vi "WPI_DashboardGet Robot IP.vi"(11 "Notifier in":refnum<notifier>) -> ()   [LabVIEW 2018]
doc: "Connect to the Driver Station to receive occasional updates including the robot IP address. Send\nnotification when you receive IP information."
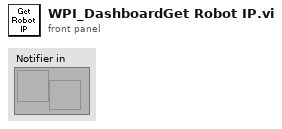
[diagram p1: front panel]
types:
  T1 = cluster{"robotIP":u32, "dashboardIP":u32, "FMS Connected":bool, "Robot Connected":bool, "RobotCode":bool}
  T2 = enum16{"Standard", "Buffered", "CRLF", "Immediate"}
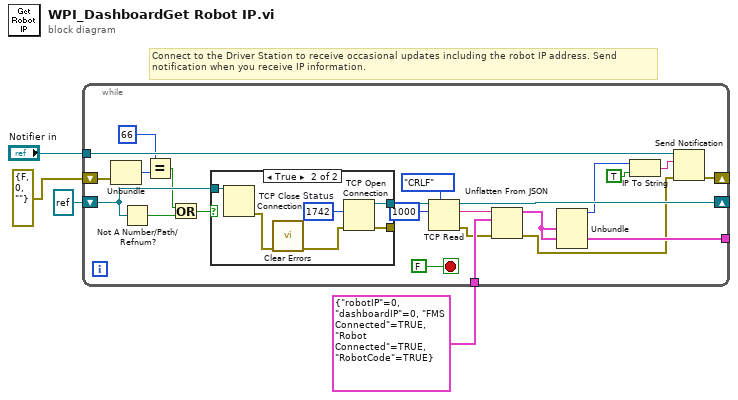
[diagram p0: block diagram]
diagram:
  # "Connect to the Driver Station to receive occasional updates including the robot IP address. Send\nnotification when you receive IP information."
  n1 = while {
    shift-right: [w22] -> _
    shift-left: refnum<k5> refnum ("connection ID") -> [w26]
    tunnel: [w18] -> _
    tunnel: T1 {"robotIP"=0, "dashboardIP"=0, "FMS Connected"=TRUE, "Robot Connected"=TRUE, "RobotCode"=TRUE} -> [w19]
    tunnel: "Notifier in" -> [w17]
    shift-right: [w11] -> _
    shift-left: errorcluster {"status"=FALSE, "code"=0, "source"=""} ("error out") -> [w8]
    stop <- FALSE stop-if-true
    n2 = Unbundle(w8) -> ("code"=w7:i32)  [unwired: 2 out]
    n3 = Not A Number/Path/Refnum?(number/path/refnum=w26) -> (NaN/Path/Refnum?=w10:bool)
    n4 = Equal?(x=66, y=w7) -> (x = y?=w5:bool)
    n5 = Or(x=w5, y=w10) -> (x .or. y?=w9:bool)
    n6 = case shown="True" w9 {
      tunnel: [w27 w32] -> w24
      tunnel: w26 -> [w27 w31]
      tunnel: [_ w30] -> _
      frame False {
      }
      frame True {
        w33 = u16 1742  # Status
        n7 = TCP Close Connection(connection ID=w31) -> (error out=w29:errorcluster)  [unwired: 2 in, 1 out]
        n8 = call <vilib>:"Clear Errors.vi"("error in (no error)"=w29) -> ("error out"=w28:errorcluster)  [unwired: 5 in, 1 out]
        n9 = TCP Open Connection(remote port or service name=w33, error in (no error)=w28) -> (connection ID=w32:refnum<k5>, error out=w30:errorcluster)  [unwired: 3 in]
      }
    }
    n10 = TCP Read(connection ID=w24, bytes to read=1000, 7:T2."CRLF" ("mode (standard)")) -> (connection ID out=w22:refnum<k5>, data out=w20:string, error out=w15:errorcluster)  [unwired: 2 in]
    n11 = Unflatten From JSON(JSON string=w20, type and defaults=w19, error in (no error)=w15) -> (value=w18:T1, error out=w12:errorcluster)  [unwired: 4 in]
    n12 = Unbundle(w18) -> ("robotIP"=w16:u32)  [unwired: 4 out]
    n13 = IP To String(1:TRUE ("dot notation? (F)"), 2:w16) -> (0:w14:string)
    n14 = Send Notification(notification=w14, notifier=w17, error in (no error)=w12) -> (error out=w11:errorcluster)  [unwired: 1 out]
  }
